vi "Update SyncMethod Event Structure.vi"(8 "error in (no error)":errorcluster, 11 "Server class in":refnum<vi>) -> (0 "error out":errorcluster, 3 "Server class out":refnum<vi>)   [LabVIEW 2019, in "gRPC Template Creation Utility.lvlib"]
uses:
  gRPC Template Creation Utility.lvlib
  <vilib>/event_ctls.llb/lveventtype.ctl
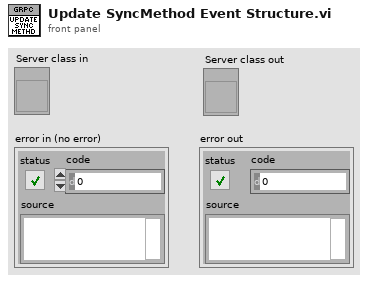
[diagram p1: front panel]
types:
  T1 = typedef "lveventtype.ctl" = enum32{"Null", "Timeout", "Annotation Menu Selection", "Annotation Menu Selection?", "App Instance Close", "App Instance Close?", "Autoscale Range Change", "Bookmark Info Change", "Cell Edit", "Cell Edit?", "Cursor Grab", "Cursor Grab?", "Cursor Menu Selection", "Cursor Menu Selection?", "Cursor Move", "Cursor Release", "Data Change", "Direction Change", "Display State Change", "Drag Ended", "Drag Enter", "Drag Leave", "Drag Over", "Drag Source Update", "Drag Starting", "Drag Starting?", "Drop", "Exec State Change", "Key Down", "Key Down?", "Key Repeat", "Key Repeat?", "Key Up", "Listbox Double Click", "Menu Activation?", "Menu Selection (App)", "Menu Selection? (App)", "Menu Selection (User)", "Mouse Down", "Mouse Down?", "Mouse Enter", "Mouse Leave", "Mouse Move", "Mouse Up", "Mouse Wheel", "NI Security User Change (App)", "Pane Size", "Panel Close", "Panel Close?", "Panel Resize", "Plot Attribute Change", "Scale Range Change", "Shortcut Menu Activation?", "Shortcut Menu Selection (App)", "Shortcut Menu Selection? (App)", "Shortcut Menu Selection (User)", "Tree Double Click", "Tree Drag", "Tree Drag?", "Tree Drop", "Tree Drop?", "Tree Item Close", "Tree Item Close?", "Tree Item Open", "Tree Item Open?", "User Event", "Value Change"}
  T2 = cluster{"Event Type":T1, "Event Registration Index":i32}
  T3 = cluster{"Event Type":T1, "Event Registration Index":i32}[]
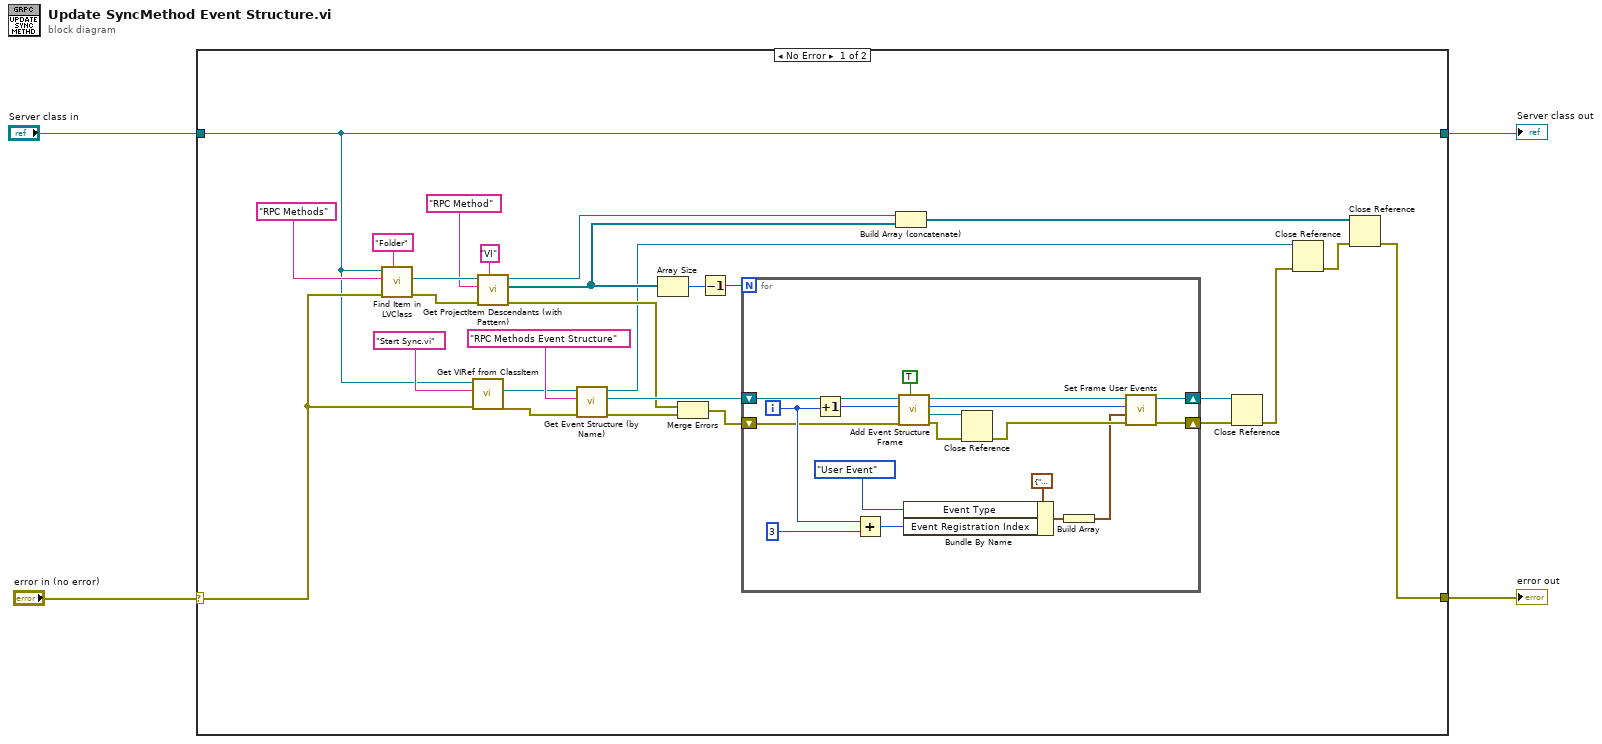
[diagram p0: block diagram]
diagram:
  n1 = case shown="No Error" "error in (no error)" {
    selector: "error in (no error)" -> [w8 w50]
    tunnel: "Server class in" -> [w7 w51]
    tunnel: [w9 w50] -> w3
    tunnel: [w7 w51] -> w1
    frame No Error {
      n2 = call "Find Item in LVClass.vi"("Item Type"="Folder", "error in (no error)"=w8, "Item Name"="RPC Methods", "Class Item in"=w7) -> ("error out"=w30:errorcluster, "Project Item (Class Item)"=w31:refnum<vi>)  [unwired: 4 in, 2 out]
      n3 = call "Get VIRef from ClassItem.vi"("error in (no error)"=w8, "Item Name"="Start Sync.vi", "LVClassLibrary in"=w7) -> ("error out"=w22:errorcluster, "VIref out"=w24:refnum<vi>)  [unwired: 5 in, 2 out]
      n4 = call "Get ProjectItem Descendants (with Pattern).vi"("Type"="VI", "error in (no error)"=w30, "Pattern"="RPC Method" ("regular expression"), "ProjectItem in"=w31) -> ("error out"=w15:errorcluster, "ProjectItem descendents"=w13:refnum<vi>[], "ProjectItem out"=w18:refnum<vi>)  [unwired: 5 in]
      n5 = call "Get Event Structure (by Name).vi"("error in (no error)"=w22, "Label"="RPC Methods Event Structure", "Owner VI in"=w24) -> ("error out"=w16:errorcluster, "Event Structure ref out"=w21:refnum<vi>, "Owner VI out"=w11:refnum<vi>)  [unwired: 5 in, 1 out]
      n6 = Array Size(array=w13) -> (size(s)=w6:i32)
      n7 = Merge Errors(w15, w16) -> (w14:errorcluster)
      n8 = Decrement(x=w6) -> (x-1=w5:i32)
      n9 = for {
        N: w5 -> [_]
        shift-right: [w35] -> w20
        shift-left: w14 -> [w33]
        shift-right: [w32] -> w19
        shift-left: w21 -> [w34]
        i -> [w40]
        n10 = Increment(x=w40) -> (x+1=w43:i32)
        n11 = Add(x=w40, y=3) -> (x+y=w38:i32)
        n12 = call "Add Event Structure Frame.vi"("After? (T)"=TRUE, "error in (no error)"=w33, "Reference Frame Index"=w43, "Event Structure ref in"=w34) -> ("error out"=w49:errorcluster, "Added Frame"=w48:refnum<vi>, "Added Frame Index"=w46:i32, "Event Structure ref out"=w45:refnum<vi>)  [unwired: 4 in]
        n13 = Bundle By Name(cluster=T2 {"Event Type"=enum."User Event", "Event Registration Index"=3} ("Dynamic Events"), "Event Type"=lveventtype."User Event", "Event Registration Index"=w38) -> (w37:T2)
        n14 = Close Reference(reference=w48, error in (no error)=w49) -> (error out=w47:errorcluster)
        n15 = Build Array(w37) -> (w36:T3)
        n16 = call "Set Frame User Events.vi"("error in (no error)"=w47, "Dynamic Events"=w36, "Frame Index in"=w46, "Event Structure ref in"=w45) -> ("error out"=w35:errorcluster, "Event Structure ref out"=w32:refnum<vi>)  [unwired: 5 in, 1 out]
      }
      n17 = Build Array (concatenate)(w18, w13) -> (w17:refnum<vi>[])
      n18 = Close Reference(reference=w19, error in (no error)=w20) -> (error out=w12:errorcluster)
      n19 = Close Reference(reference=w11, error in (no error)=w12) -> (error out=w10:errorcluster)
      n20 = Close Reference(reference=w17, error in (no error)=w10) -> (error out=w9:errorcluster)
    }
    frame Error {
    }
  }
  "error out" <- w3
  "Server class out" <- w1
